vi "Demo_SerialProcessorTest.vi"() -> ()   [LabVIEW 2016]
uses:
  SerialSupport/Serial - Settings.ctl
  SerialSupport/Serial - XON-XOFF Characters.ctl
  SerialSupport/Serial - ASCII Characters.ctl
  <vilib>/Instr/_visa.llb/VISA Configure Serial Port (Instr).vi
  database/database.lvlib
panel:
  in  "总压降":dbl
  in  "参考电阻":dbl
  in  "JSON parser":T1
  in  "TestId":string
  out "波形图表 2":dynamicdata(graph)
  out "json error":errorcluster caption="JSON Error"
  in  "dataLabel":string
  in  "msg_id":dbl
  out "CtrlCmdMsg":string
  out "串口信息发送持久化":bool=TRUE
  out "串口信息发送":bool=TRUE
  out "UDP发送持久化":bool=TRUE
  out "TCP发送持久化":bool=TRUE
  out "串口接收持久化":bool=TRUE
  in  "串口发送按钮":bool
  in  "终止符":u8=10 format="%.0x"
  in  "终止符时结束写入？":bool=TRUE
  in  "VISA资源名称":refnum<visa-resource-name>="COM10"
  in  "XON/XOFF字符":T2={"XON"=enum."DC1", "XOFF"=enum."DC3"}
  in  "串口设置":T4={"波特率"=115200, "数据位"=8, "校验"=enum."None", "停止位"=10, "流控制"=0} {"流控制" items=["无"=0, "XON/XOFF"=1, "RTS/CTS"=2, "DTR/DSR"=4]; "停止位" items=["1.0"=10, "1.5"=15, "2.0"=20]; "数据位" min=5 max=8 step=1; "波特率" items=["75"=75, "110"=110, "134"=134, "150"=150, "300"=300, "600"=600, "1200"=1200, "1800"=1800, "2400"=2400, "4800"=4800, "7200"=7200, "9600"=9600, "14400"=14400, "19200"=19200, "28800"=28800, "38400"=38400, "56000"=56000, "57600"=57600, "115200"=115200, "128000"=128000, "230400"=230400]}
  in  "终止符时结束读取？":bool=TRUE
  in  "读取":bool=TRUE
  in  "串口停止":bool
  in  "串口发送命令":string="{\"cmd\":\"CT_ON\",\"id\":\"C_FR\",on:true}"
  out "串口信息":string
  in  "串口最大字节":u32=1000
  out "当前指令":string
  # "Smart thermalchromic window monitoring"
  # "Test Information Setting"
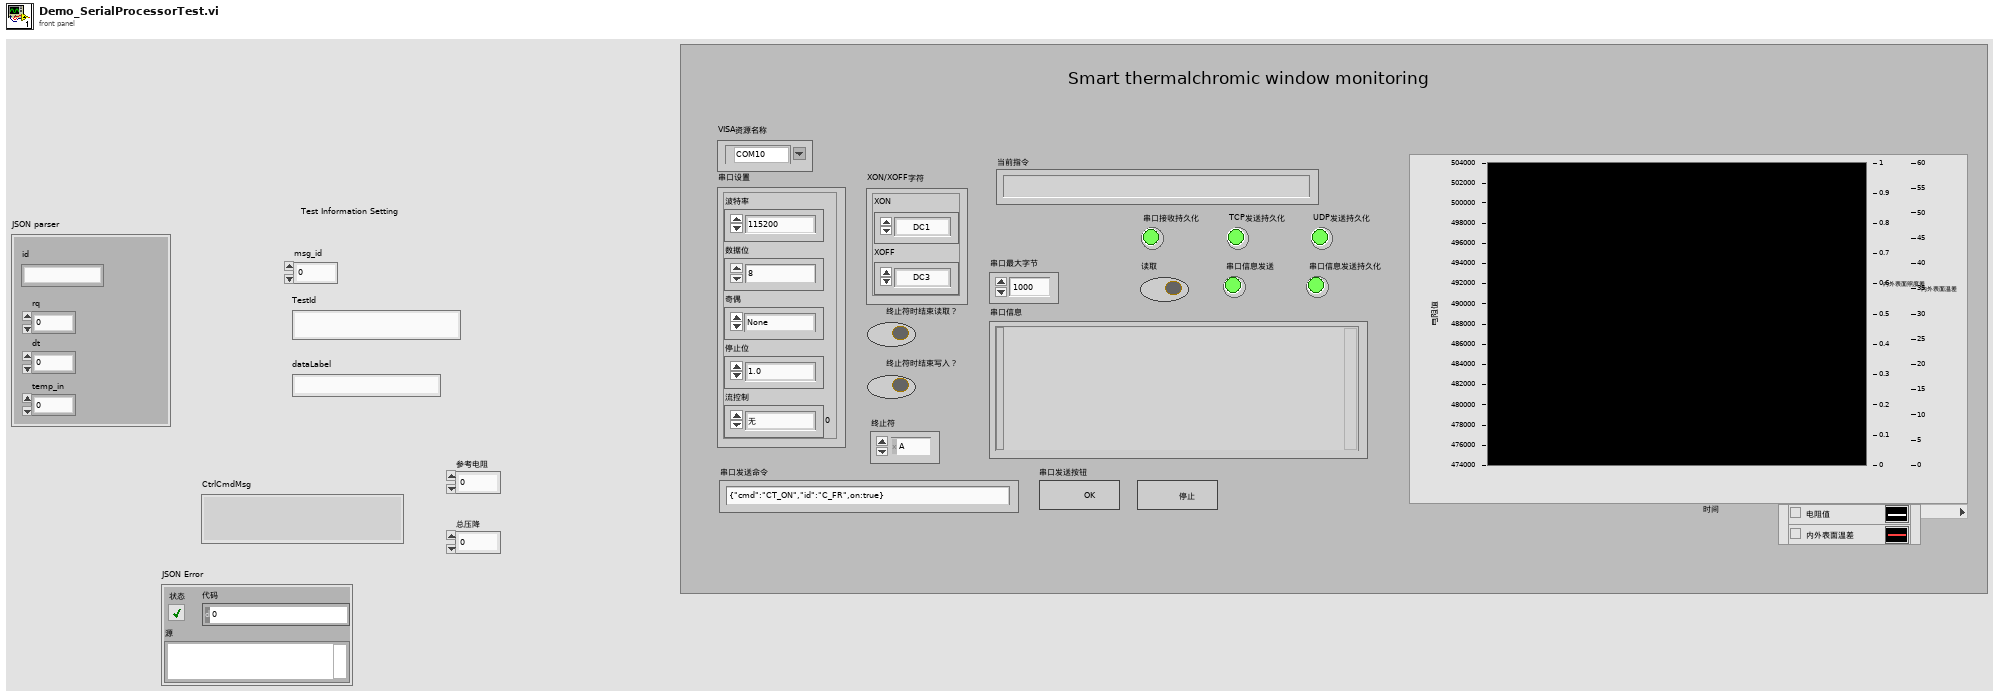
[diagram p1: front panel]
types:
  T1 = cluster{"id":string, "rq":dbl, "dt":dbl, "temp_in":dbl}
  T2 = typedef "Serial - XON-XOFF Characters.ctl" = cluster{"XON":T3, "XOFF":T3}
  T3 = typedef "Serial - ASCII Characters.ctl" = enum16{"NUL", "SOH", "STX", "ETX", "EOT", "ENQ", "ACK", "BEL", "BS", "HT", "LF", "VT", "FF", "CR", "SO", "SI", "DLE", "DC1", "DC2", "DC3", "DC4", "NAK", "SYN", "ETB", "CAN", "EM", "SUB", "ESC", "FS", "GS", "RS", "US", "SP", "!", "\"", "#", "$", "%", "&", "'", "(", ")", "*", "+", ",", "- (-)", ".", "/", "0", "1", "2", "3", "4", "5", "6", "7", "8", "9", ":", ";", "<", "=", ">", "?", "@", "A", "B", "C", "D", "E", "F", "G", "H", "I", "J", "K", "L", "M", "N", "O", "P", "Q", "R", "S", "T", "U", "V", "W", "X", "Y", "Z", "[", "\\", "]", "^", "_", "`", "a", "b", "c", "d", "e", "f", "g", "h", "i", "j", "k", "l", "m", "n", "o", "p", "q", "r", "s", "t", "u", "v", "w", "x", "y", "z", "{", "|", "}", "~"}
  T4 = typedef "Serial - Settings.ctl" = cluster{"波特率":u32, "数据位":u16, "校验":enum16{"None", "Odd", "Even", "Mark", "Space"}, "停止位":u16, "流控制":u16}
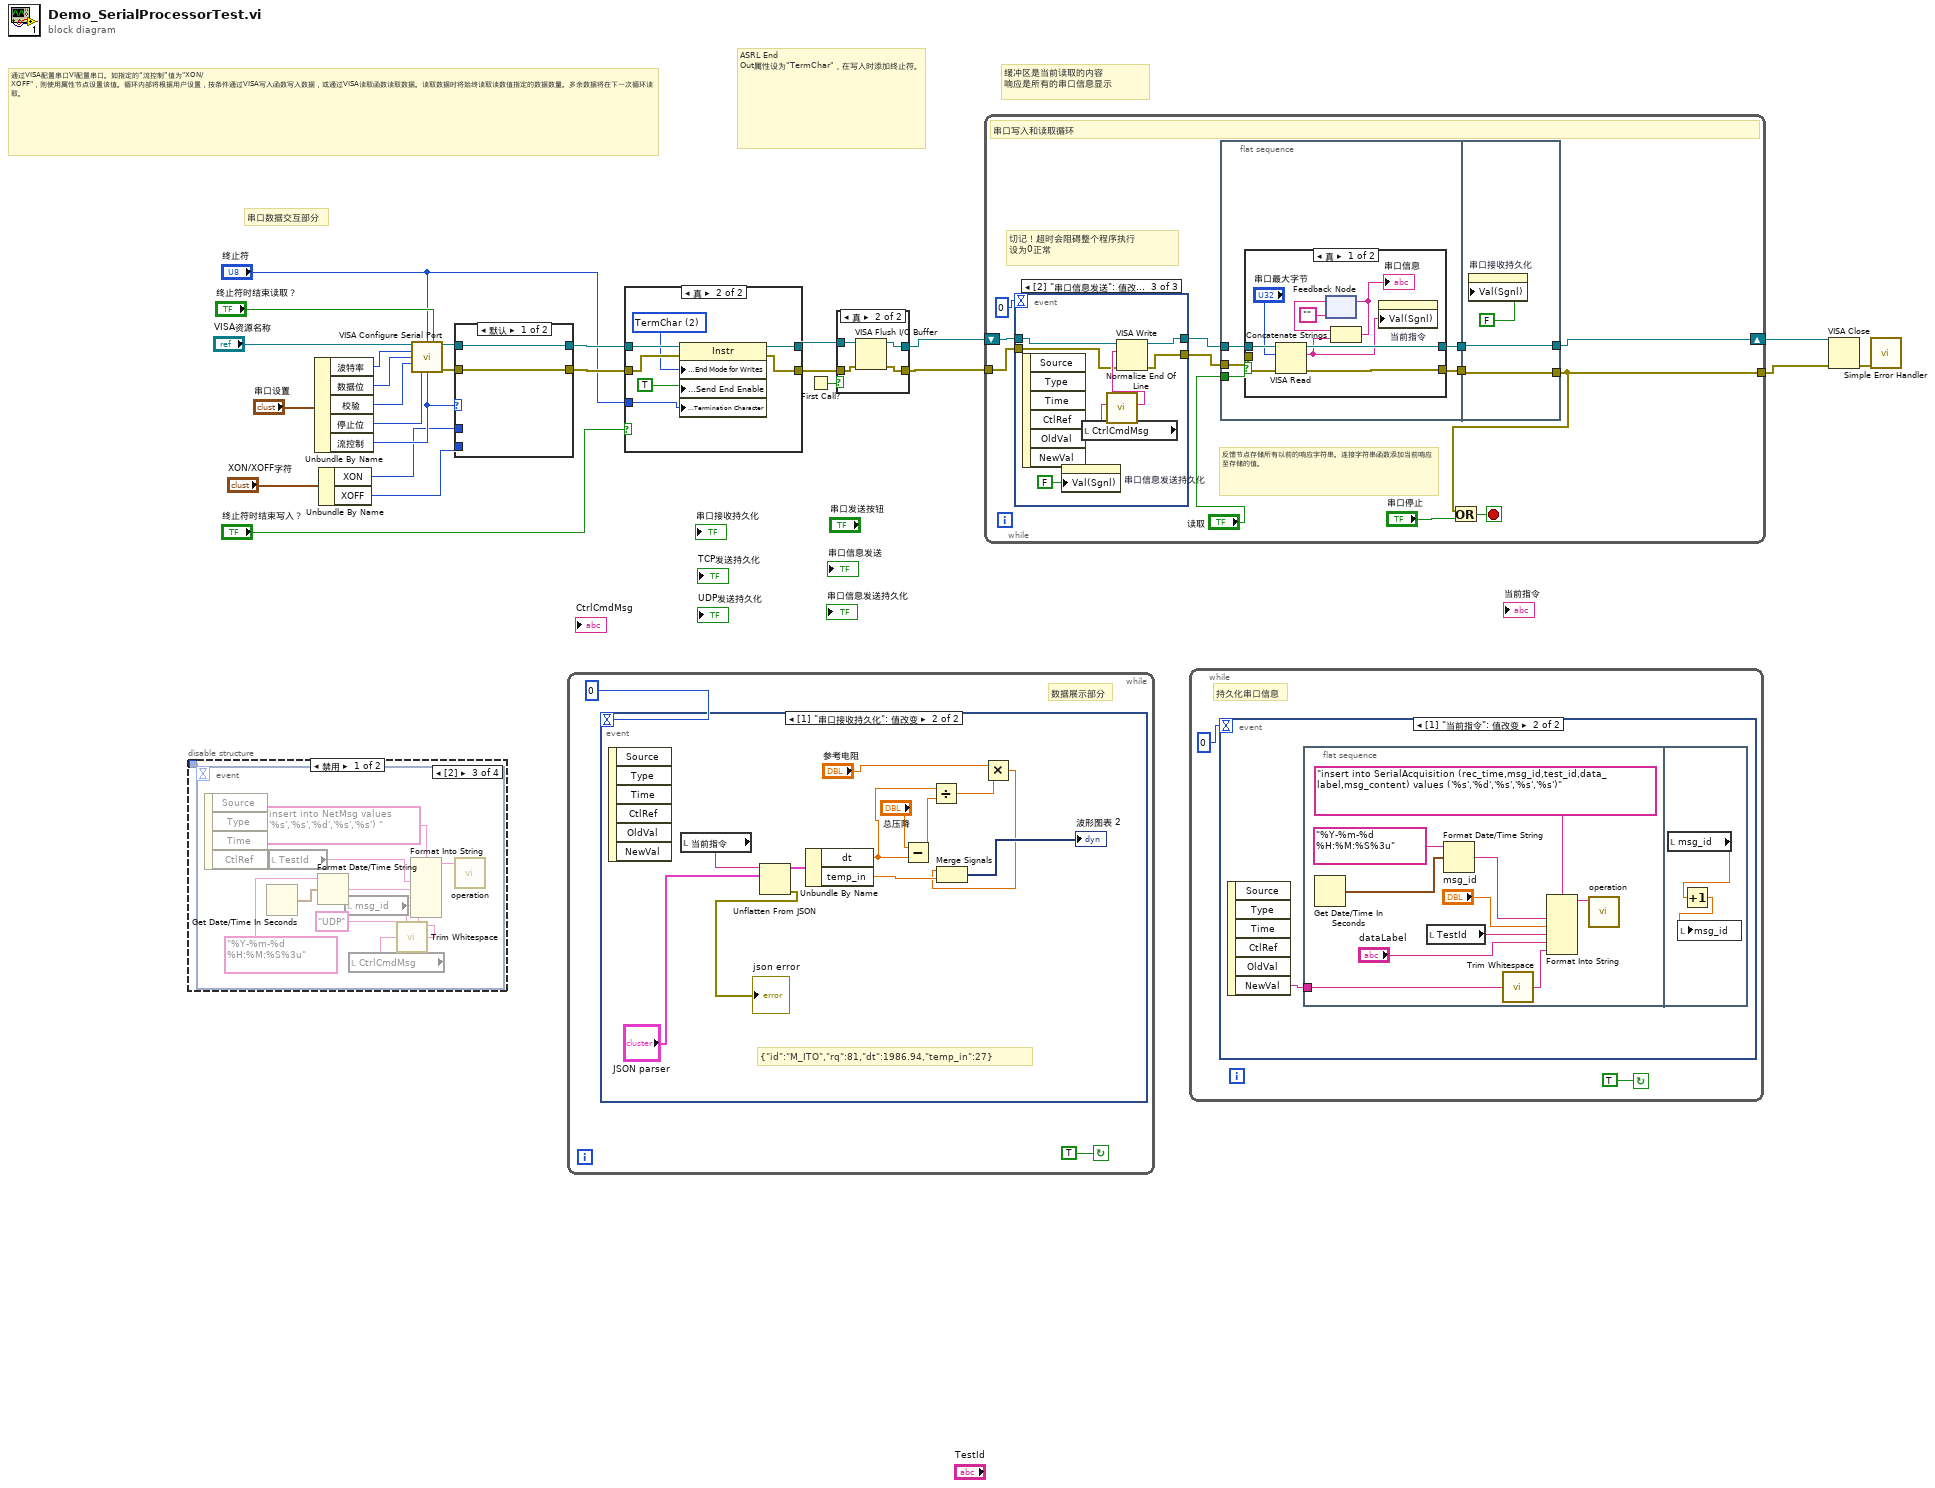
[diagram p0: block diagram]
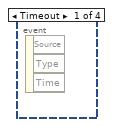
[diagram p2: hidden frame]
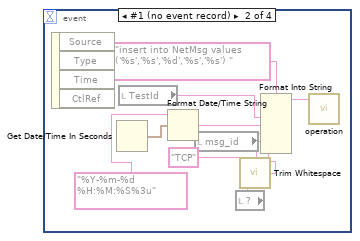
[diagram p3: hidden frame]
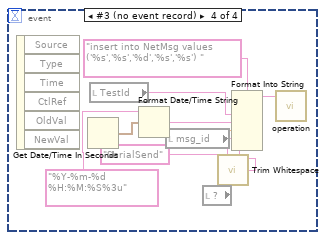
[diagram p4: hidden frame]
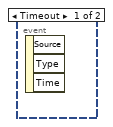
[diagram p6: hidden frame]
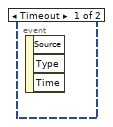
[diagram p7: hidden frame]
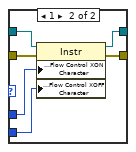
[diagram p10: hidden frame]
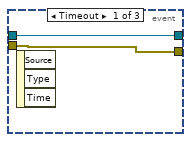
[diagram p12: hidden frame]
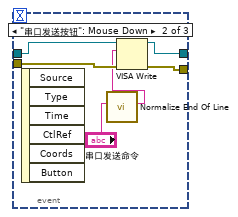
[diagram p13: hidden frame]
diagram:
  # "串口数据交互部分"
  # "缓冲区是当前读取的内容\n响应是所有的串口信息显示"
  # "ASRL End Out属性设为\"TermChar\"，在写入时添加终止符。"
  # "通过VISA配置串口VI配置串口。如指定的“流控制”值为\"XON/XOFF\"，则使用属性节点设置该值。循环内部将根据用户设置，按条件通过VISA写入函数写入数据，或通过VISA读取函数读取数据。读取数据时将始终读取读数值指定的数据数量。多余数据将在下一次循环读取。"
  n1 = disable-structure shown="禁用" {
    disable-tunnel: _ -> [w26 _]
    frame Disabled {
      n2 = event shown="[2]" {
        selector: _ -> [_ _ _ _]
        dyn-events: _ -> [_ _ _ _]
        timeout: w26 -> [_ _ _ _]
        event Timeout {
          n3 = event-data() -> ()  [unwired: 1 in, 3 out]
        }
        event #1 (no event record) {
          n4 = event-data() -> ()  [unwired: 1 in, 4 out]
          n5 = Get Date/Time In Seconds() -> (seconds since 1Jan1904=w33:timestamp)
          n6 = local read "TestId"() -> (w34:string)
          n7 = Format Date/Time String ("格式化日期/时间字符串")(time format string (%c)="%Y-%m-%d %H:%M:%S%3u" ("时间格式字符串(%c)"), seconds (now)=w33) -> (date/time string=w32:string)  [unwired: 1 in]
          n8 = local read "msg_id"() -> (w31:dbl)
          n9 = local read item#-1() -> (w28)
          n10 = call <vilib>:"Trim Whitespace.vi"("string"=w28) -> ("trimmed string"=w27:string)  [unwired: 1 in]
          n11 = Format Into String(format string="insert into NetMsg values ('%s','%s','%d','%s','%s') " ("格式字符串"), w34, w32, w31, "TCP" ("input 4"), w27) -> (resulting string=w35:string)  [unwired: 2 in, 1 out]
          n12 = call "operation.vi"("Command Text"=w35) -> ()  [unwired: 9 in, 1 out]
        }
        event #2 (no event record) {
          n13 = event-data() -> ()  [unwired: 1 in, 4 out]
          n14 = Get Date/Time In Seconds() -> (seconds since 1Jan1904=w43:timestamp)
          n15 = local read "TestId"() -> (w41:string)
          n16 = Format Date/Time String ("格式化日期/时间字符串")(time format string (%c)="%Y-%m-%d %H:%M:%S%3u" ("时间格式字符串(%c)"), seconds (now)=w43) -> (date/time string=w44:string)  [unwired: 1 in]
          n17 = local read "msg_id"() -> (w45:dbl)
          n18 = local read "CtrlCmdMsg"() -> (w38:string)
          n19 = call <vilib>:"Trim Whitespace.vi"("string"=w38) -> ("trimmed string"=w37:string)  [unwired: 1 in]
          n20 = Format Into String(format string="insert into NetMsg values ('%s','%s','%d','%s','%s') " ("格式字符串"), w41, w44, w45, "UDP" ("input 4"), w37) -> (resulting string=w40:string)  [unwired: 2 in, 1 out]
          n21 = call "operation.vi"("Command Text"=w40) -> ()  [unwired: 9 in, 1 out]
        }
        event #3 (no event record) {
          n22 = event-data() -> ()  [unwired: 1 in, 6 out]
          n23 = Get Date/Time In Seconds() -> (seconds since 1Jan1904=w53:timestamp)
          n24 = local read "TestId"() -> (w52:string)
          n25 = Format Date/Time String ("格式化日期/时间字符串")(time format string (%c)="%Y-%m-%d %H:%M:%S%3u" ("时间格式字符串(%c)"), seconds (now)=w53) -> (date/time string=w54:string)  [unwired: 1 in]
          n26 = local read "msg_id"() -> (w55:dbl)
          n27 = local read item#-1() -> (w49)
          n28 = call <vilib>:"Trim Whitespace.vi"("string"=w49) -> ("trimmed string"=w48:string)  [unwired: 1 in]
          n29 = Format Into String(format string="insert into NetMsg values ('%s','%s','%d','%s','%s') " ("格式字符串"), w52, w54, w55, "SerialSend" ("input 4"), w48) -> (resulting string=w51:string)  [unwired: 2 in, 1 out]
          n30 = call "operation.vi"("Command Text"=w51) -> ()  [unwired: 9 in, 1 out]
        }
      }
    }
    frame Enabled {
    }
  }
  n31 = Unbundle By Name("串口设置") -> ("波特率"=w18:u32, "数据位"=w19:u16, "校验"=w20:enum16{"None", "Odd", "Even", "Mark", "Space"}, "停止位"=w21:u16, "流控制"=w13:u16)
  n32 = Unbundle By Name("XON/XOFF字符") -> ("XON"=w12:T3, "XOFF"=w11:T3)
  n33 = call-poly "VISA Configure Serial Port"("VISA resource name"="VISA资源名称", "termination char\n(0xA = '\\n' = LF)"="终止符", "Enable Termination\nChar (T)"="终止符时结束读取？", "baud rate (9600)"=w18, "data bits (8)"=w19, "parity (0:none)"=w20, "stop bits (10: 1 bit)"=w21, "flow control (0:none)"=w13) -> ("VISA resource name out"=w22:refnum<visa-resource-name>, "error out"=w23:errorcluster)  [unwired: 2 in, 4 out]
  n34 = case shown="默认" w13 {
    tunnel: [w57 w64] -> w10
    tunnel: [w58 w63] -> w9
    tunnel: w23 -> [w57 w62]
    tunnel: w22 -> [w58 w61]
    tunnel: w12 -> [_ w60]
    tunnel: w11 -> [_ w59]
    frame Default {
    }
    frame 1 {
      n35 = property class="Instr"(reference=w61, error in=w62, "Serial Settings:Flow Control XON Character"=w60, "Serial Settings:Flow Control XOFF Character"=w59) -> (reference out=w63:refnum<visa-resource-name>, error out=w64:errorcluster)
    }
  }
  n36 = while {
    stop <- TRUE continue-if-true
    # "数据展示部分"
    n37 = event shown="[1] \"串口接收持久化\": 值改变" {
      selector: _ -> [_ _]
      dyn-events: _ -> [_ _]
      timeout: 0 -> [_ _]
      event Timeout {
        n38 = event-data() -> ()  [unwired: 1 in, 3 out]
      }
      event "串口接收持久化": Value Change {
        # "{\"id\":\"M_ITO\",\"rq\":81,\"dt\":1986.94,\"temp_in\":27}"
        n39 = event-data() -> ()  [unwired: 1 in, 6 out]
        n40 = local read "当前指令"() -> (w78:string)
        n41 = Unflatten From JSON(JSON string=w78, type and defaults="JSON parser") -> (value=w75:T1, error out=→"json error":errorcluster)  [unwired: 5 in]
        n42 = Unbundle By Name(w75) -> ("dt"=w71:dbl, "temp_in"=w74:dbl)
        n43 = Subtract(x="总压降", y=w71) -> (x-y=w70:dbl)
        n44 = Divide(x=w71, y=w70) -> (x/y=w69:dbl)
        n45 = Multiply(x="参考电阻", y=w69) -> (x*y=w67:dbl)
        n46 = Merge Signals(w67, w74) -> (→"波形图表 2":dynamicdata)
      }
    }
  }
  n47 = case shown="真" "终止符时结束写入？" {
    tunnel: w9 -> [w79 w87]
    tunnel: w10 -> [w80 w86]
    tunnel: [w79 w85] -> w6
    tunnel: [w80 w84] -> w5
    tunnel: "终止符" -> [_ w82]
    frame False {
    }
    frame True {
      w83 = u16 2 items=["None", "LastBit", "TermChar", "Break"] ("Serial Settings:Serial End Mode for Writes")
      n48 = property class="Instr"(reference=w87, error in=w86, "Serial Settings:End Mode for Writes"=w83, "Message Based Settings:Send End Enable"=TRUE, "Message Based Settings:Termination Character"=w82) -> (reference out=w85:refnum<visa-resource-name>, error out=w84:errorcluster)
    }
  }
  n49 = First Call?() -> (First Call?: T/F=w2:bool)
  n50 = case shown="真" w2 {
    tunnel: w6 -> [w89 w93]
    tunnel: w5 -> [w88 w92]
    tunnel: [w89 w91] -> w4
    tunnel: [w88 w90] -> w3
    frame False {
    }
    frame True {
      n51 = VISA Flush I/O Buffer(VISA resource name=w93, error in (no error)=w92) -> (VISA resource name out=w91:refnum<visa-resource-name>, error out=w90:errorcluster)  [unwired: 1 in]
    }
  }
  n52 = while {
    shift-right: [w95] -> w14
    shift-left: w4 -> [w100]
    tunnel: w3 -> [w102]
    tunnel: [w94] -> w1
    stop <- w104 stop-if-true
    # "反馈节点存储所有以前的响应字符串。连接字符串函数添加当前响应至存储的值。"
    # "切记！超时会阻碍整个程序执行\n设为0正常"
    # "串口写入和读取循环"
    n53 = event shown="[2] \"串口信息发送\": 值改变" {
      selector: _ -> [_ _ _]
      dyn-events: _ -> [_ _ _]
      timeout: 0 -> [_ _ _]
      tunnel: w102 -> [w125 w132 w135]
      tunnel: [w125 w131 w136] -> w101
      tunnel: w100 -> [w126 w130 w138]
      tunnel: [w126 w129 w137] -> w99
      event Timeout {
        n54 = event-data() -> ()  [unwired: 1 in, 3 out]
      }
      event "串口发送按钮": Mouse Down {
        n55 = event-data() -> ()  [unwired: 1 in, 6 out]
        n56 = call <vilib>:"Normalize End Of Line.vi"("string in"="串口发送命令") -> ("string out"=w127:string)  [unwired: 7 in]
        n57 = VISA Write(VISA resource name=w130, write buffer=w127, error in (no error)=w132) -> (VISA resource name out=w129:refnum<visa-resource-name>, error out=w131:errorcluster)  [unwired: 1 out]
      }
      event "串口信息发送": Value Change {
        n58 = event-data() -> ()  [unwired: 1 in, 6 out]
        n59 = property on="串口信息发送持久化" class="Bool (严格)"("Val(Sgnl)"=FALSE ("Value (Signaling)")) -> ()  [unwired: 2 in, 2 out]
        n60 = local read "CtrlCmdMsg"() -> (w134:string)
        n61 = call <vilib>:"Normalize End Of Line.vi"("string in"=w134) -> ("string out"=w139:string)  [unwired: 7 in]
        n62 = VISA Write(VISA resource name=w138, write buffer=w139, error in (no error)=w135) -> (VISA resource name out=w137:refnum<visa-resource-name>, error out=w136:errorcluster)  [unwired: 1 out]
      }
    }
    n63 = flat-sequence {
      tunnel: "读取" -> [w109]
      tunnel: w101 -> [w107]
      tunnel: w99 -> [w106]
      tunnel: [w110] -> w97
      tunnel: [w108] -> w96
      tunnel: w97 -> [w123]
      tunnel: w96 -> [w122]
      tunnel: [w123] -> w95
      tunnel: [w122] -> w94
      frame #0 {
        n64 = case shown="真" w109 {
          tunnel: [w117 w121] -> w110
          tunnel: w106 -> [w119 w121]
          tunnel: [w115 w120] -> w108
          tunnel: w107 -> [w118 w120]
          frame True {
            n65 = VISA Read(VISA resource name=w119, byte count="串口最大字节", error in (no error)=w118) -> (VISA resource name out=w117:refnum<visa-resource-name>, read buffer=w111:string, error out=w115:errorcluster)  [unwired: 1 out]
            n66 = feedback #1("") -> (w114:string)
            n67 = Concatenate Strings(w114, w111) -> (w113:string)
            "串口信息" <- w113
            n68 = feedback-in #1(w113) -> ()
            n69 = property on="当前指令" class="Str"("Val(Sgnl)"=w111) -> ()  [unwired: 2 in, 2 out]
          }
          frame False {
          }
        }
      }
      frame #1 {
        n70 = property on="串口接收持久化" class="Bool (严格)"("Val(Sgnl)"=FALSE ("Value (Signaling)")) -> ()  [unwired: 2 in, 2 out]
      }
    }
    n71 = Or(x=w94, y="串口停止") -> (x .or. y?=w104:bool)
  }
  n72 = while {
    stop <- TRUE continue-if-true
    # "持久化串口信息"
    n73 = event shown="[1] \"当前指令\": 值改变" {
      selector: _ -> [_ _]
      dyn-events: _ -> [_ _]
      timeout: 0 -> [_ _]
      event Timeout {
        n74 = event-data() -> ()  [unwired: 1 in, 3 out]
      }
      event "当前指令": Value Change {
        n75 = event-data() -> ("NewVal"=w142:string)  [unwired: 1 in, 5 out]
        n76 = flat-sequence {
          tunnel: w142 -> [w144]
          frame #0 {
            n77 = Get Date/Time In Seconds() -> (seconds since 1Jan1904=w150:timestamp)
            n78 = local read "TestId"() -> (w146:string)
            n79 = Format Date/Time String ("格式化日期/时间字符串")(time format string (%c)="%Y-%m-%d %H:%M:%S%3u" ("时间格式字符串(%c)"), seconds (now)=w150) -> (date/time string=w147:string)  [unwired: 1 in]
            n80 = call <vilib>:"Trim Whitespace.vi"("string"=w144) -> ("trimmed string"=w148:string)  [unwired: 1 in]
            n81 = Format Into String(format string="insert into SerialAcquisition (rec_time,msg_id,test_id,data_label,msg_content) values ('%s','%d','%s','%s','%s')" ("格式字符串"), w147, "msg_id", w146, "dataLabel", w148) -> (resulting string=w149:string)  [unwired: 2 in, 1 out]
            n82 = call "operation.vi"("Command Text"=w149) -> ()  [unwired: 9 in, 1 out]
          }
          frame #1 {
            n83 = local read "msg_id"() -> (w154:dbl)
            n84 = Increment(x=w154) -> (x+1=w153:dbl)
            n85 = local write "msg_id"(w153) -> ()
          }
        }
      }
    }
  }
  n86 = VISA Close(VISA resource name=w14, error in (no error)=w1) -> (error out=w15:errorcluster)
  n87 = call <vilib>:"Simple Error Handler.vi"("error in (no error)"=w15) -> ()  [unwired: 1 in, 8 out]
